vi "get name from function.vi"(7 "owner":string, 10 "processing function":T1, 11 "engine configuration in":refnum<class "engine configuration.lvclass">) -> (2 "name":string, 3 "engine configuration out":refnum<class "engine configuration.lvclass">)   [LabVIEW 2013, in "tag bus processing plugin module configuration.lvclass"]
uses:
  tag bus processing plugin module configuration.lvclass
  processing channels.ctl
  <vilib>/NI/Tag Bus Module Framework/channel/TBM channel.lvclass
  <vilib>/NI/Module Execution Interface/Engine Configuration/engine configuration.lvclass
  <vilib>/NI/Tag Bus/tag/tag descriptor.lvclass/tag descriptor.ctl
  <vilib>/NI/Tag Bus/tag/tag descriptor.lvclass
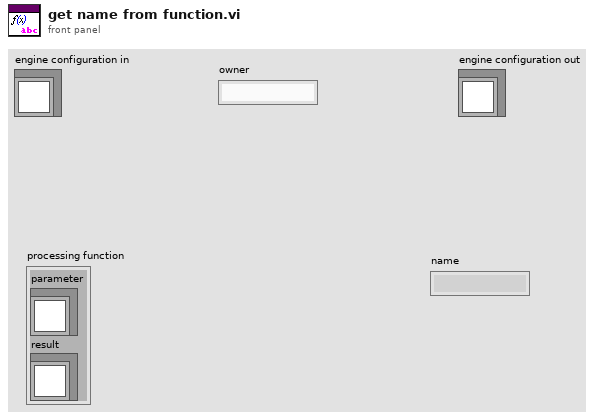
[diagram p1: front panel]
types:
  T1 = typedef "tag bus processing plugin module configuration.lvclass/processing channels.ctl" = cluster{"parameter":refnum<class "TBM channel.lvclass">, "result":refnum<class "TBM channel.lvclass">}
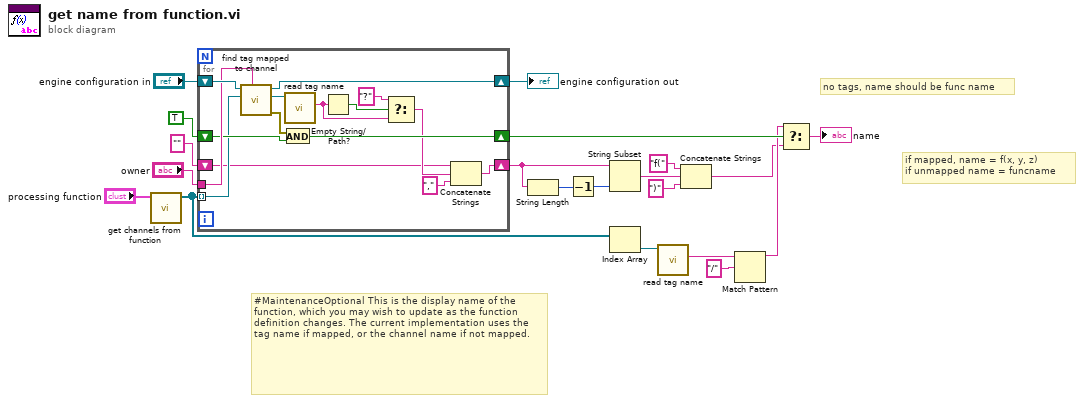
[diagram p0: block diagram]
diagram:
  # "#MaintenanceOptional This is the display name of the function, which you may wish to update as the function definition changes. The current implementation uses the tag name if mapped, or the channel name if not mapped."
  # "if mapped, name = f(x, y, z)\nif unmapped name = funcname"
  # "no tags, name should be func name"
  n1 = call "get channels from function.vi"("processing function"="processing function") -> ("channels"=w15:refnum<class "TBM channel.lvclass">[])  [unwired: 10 in]
  n2 = for {
    shift-right: [w34] -> w17
    shift-left: "engine configuration in" -> [w35]
    tunnel: "owner" -> [w33]
    shift-right: [w31] -> w11
    shift-left: TRUE -> [w30]
    tunnel: w15 -> [w29] mode=indexing
    shift-right: [w22] -> w4
    shift-left: "" -> [w21]
    n3 = call <vilib>:"find tag mapped to channel.vi"("owner"=w33, "channel"=w29, "engine configuration in"=w35) -> ("error out"=w32:errorcluster, "tag"=w28:refnum<class "tag descriptor.lvclass">, "engine configuration out"=w34:refnum<class "engine configuration.lvclass">)  [unwired: 6 in]
    n4 = And(x=w32, y=w30) -> (x .and. y?=w31:bool)
    n5 = call <vilib>:"read tag name.vi"("system tag in"=w28) -> ("name"=w26:string)  [unwired: 8 in, 2 out]
    n6 = Empty String/Path?(string/path=w26) -> (empty?=w27:bool)
    n7 = Select(t="?", s=w27, f=w26) -> (s? t:f=w24:string)
    n8 = Concatenate Strings(w21, w24, "," ("string")) -> (w22:string)
  }
  "engine configuration out" <- w17
  n9 = String Length(string=w4) -> (length=w3:i32)
  n10 = Decrement(x=w3) -> (x-1=w2:i32)
  n11 = String Subset(string=w4, length (rest)=w2) -> (substring=w1:string)  [unwired: 1 in]
  n12 = Index Array(array=w15) -> (element=w14:refnum<class "TBM channel.lvclass">)  [unwired: 1 in]
  n13 = call <vilib>:"read tag name.vi"("system tag in"=w14) -> ("name"=w13:string)  [unwired: 8 in, 2 out]
  n14 = Concatenate Strings("f(", w1, ")") -> (w6:string)
  n15 = Match Pattern(string=w13, regular expression="/") -> (before substring=w10:string)  [unwired: 1 in, 3 out]
  n16 = Select(t=w10, s=w11, f=w6) -> (s? t:f=→"name":string)
